vi "Series_ejes_flota.vi"(5 "Tabla_flota":string[][](array[string]), 6 "Tags":string[](array[string])) -> (0 "Nº Ejes":i32[](array[numeric]), 1 "Series del convoy":string[](array[string]), 4 "UT":i32[](array[numeric]))   [LabVIEW 2015]
panel:
  out "Array 2":i32[](array[numeric])
  out "Array":i32[](array[numeric])
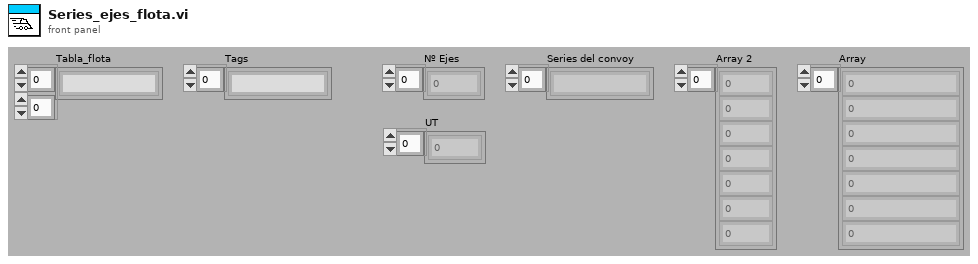
[diagram p1: front panel]
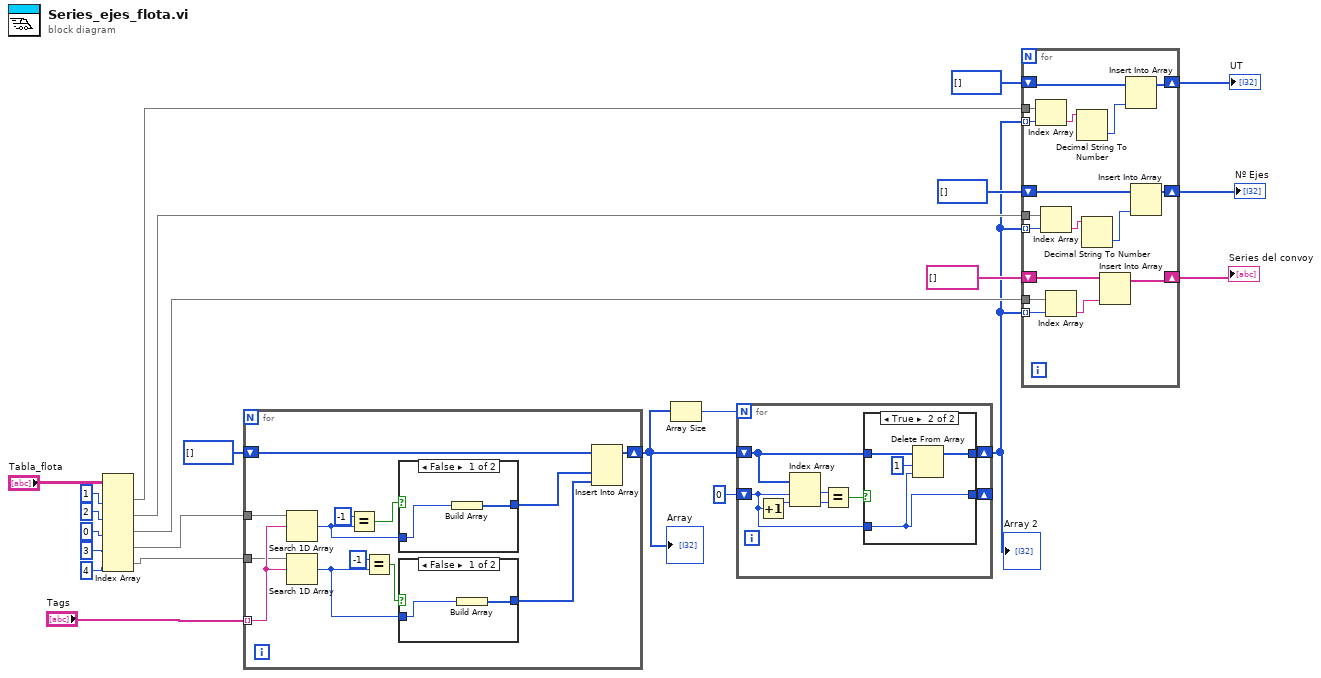
[diagram p0: block diagram]
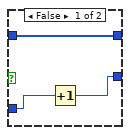
[diagram p2: hidden frame]
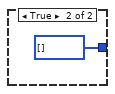
[diagram p3: hidden frame]
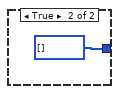
[diagram p4: hidden frame]
diagram:
  n1 = Index Array(array="Tabla_flota", index (col) #1=1 ("index (row)"), index (col) #2=2 ("disabled index (col)"), index (col) #3=0 ("disabled index (col)"), index (col) #4=3 ("disabled index (col)"), index (col) #5=4 ("index (col)")) -> (element #1=w4:string[], element #2=w20:string[], element #3=w17:string[], element #4=w10:string[], element #5=w11:string[])  [unwired: 5 in]
  n2 = for {
    tunnel: "Tags" -> [w36] mode=indexing
    tunnel: w10 -> [w35]
    tunnel: w11 -> [w34]
    shift-right: [w32] -> w13
    shift-left: i32[] [] -> [w33]
    n3 = Search 1D Array(1D array=w35, element=w36) -> (index of element=w25:i32)  [unwired: 1 in]
    n4 = Search 1D Array(1D array=w34, element=w36) -> (index of element=w24:i32)  [unwired: 1 in]
    n5 = Equal?(x=-1, y=w25) -> (x = y?=w29:bool)
    n6 = Equal?(x=-1, y=w24) -> (x = y?=w28:bool)
    n7 = case shown="False" w29 {
      tunnel: [w40 i32[] []] -> w27
      tunnel: w25 -> [w41 _]
      frame False {
        n8 = Build Array(w41) -> (w40:i32[])
      }
      frame True {
      }
    }
    n9 = case shown="False" w28 {
      tunnel: [w37 i32[] []] -> w26
      tunnel: w24 -> [w38 _]
      frame False {
        n10 = Build Array(w38) -> (w37:i32[])
      }
      frame True {
      }
    }
    n11 = Insert Into Array(array=w33, new element #1=w27, new element #2=w26) -> (w32:i32[])  [unwired: 1 in]
  }
  "Array" <- w13
  n12 = Array Size(array=w13) -> (size(s)=w15:i32)
  n13 = for {
    N: w15 -> [_]
    shift-right: [w46] -> w3
    shift-left: w13 -> [w47]
    shift-right: [w43] -> _
    shift-left: 0 -> [w44]
    n14 = Increment(x=w44) -> (x+1=w45:i32)
    n15 = Index Array(array=w47, index #1=w44, index #2=w45) -> (element #1=w49:i32, element #2=w50:i32)
    n16 = Equal?(x=w49, y=w50) -> (x = y?=w48:bool)
    n17 = case shown="True" w48 {
      tunnel: w47 -> [w53 w57]
      tunnel: [w53 w56] -> w46
      tunnel: w44 -> [w52 w54]
      tunnel: [w51 w54] -> w43
      frame False {
        n18 = Increment(x=w52) -> (x+1=w51:i32)
      }
      frame True {
        n19 = Delete From Array(array=w57, length=1, index=w54) -> (array with subset deleted=w56:i32[])  [unwired: 1 out]
      }
    }
  }
  "Array 2" <- w3
  n20 = for {
    tunnel: w3 -> [w74] mode=indexing
    tunnel: w17 -> [w73]
    shift-right: [w70] -> w23
    shift-left: string[] [] -> [w71]
    tunnel: w20 -> [w69]
    tunnel: w3 -> [w68] mode=indexing
    shift-right: [w66] -> w22
    shift-left: i32[] [] -> [w67]
    shift-right: [w60] -> w2
    shift-left: i32[] [] -> [w61]
    tunnel: w4 -> [w59]
    tunnel: w3 -> [w58] mode=indexing
    n21 = Index Array(array=w59, index=w58) -> (element=w63:string)
    n22 = Index Array(array=w69, index=w68) -> (element=w65:string)
    n23 = Index Array(array=w73, index=w74) -> (element=w72:string)
    n24 = Decimal String To Number(string=w63) -> (number=w62:i32)  [unwired: 2 in, 1 out]
    n25 = Decimal String To Number(string=w65) -> (number=w64:i32)  [unwired: 2 in, 1 out]
    n26 = Insert Into Array(array=w71, new element=w72) -> (w70:string[])  [unwired: 1 in]
    n27 = Insert Into Array(array=w61, new element=w62) -> (w60:i32[])  [unwired: 1 in]
    n28 = Insert Into Array(array=w67, new element=w64) -> (w66:i32[])  [unwired: 1 in]
  }
  "Series del convoy" <- w23
  "Nº Ejes" <- w22
  "UT" <- w2
